vi "MODBUS_read_register.vi"(5 "Byte order":T1(ring)=enum."2-3-0-1", 6 "data type":enum16{"float", "UINT", "UINT32", "STRING"}(ring)=enum."STRING", 7 "MODBUS Serial Parameters":T3={"Mode"=enum."RTU", "Default Slave Address"=111, "MODBUS timeout"=1000, "Baud Rate"=38400, "Parity"=0, "Flow Control"=0} {"Parity" items=["None", "Odd", "Even", "Mark", "Space"]; "Flow Control" items=["None", "XON/XOFF", "RTS/CTS", "XON/XOFF & RTS/CTS", "DTR/DSR", "XON/XOFF & DTR/DSR"]}, 8 "error in":errorcluster, 9 "Register":u16=285, 10 "Length":u16=1, 11 "VISA resource name":refnum<visa-resource-name>="MODBUS_485") -> (0 "error out":errorcluster, 1 "found?":bool, 2 "output cluster":T2, 3 "VISA resource name out":refnum<visa-resource-name>)   [LabVIEW 2016]
uses:
  NI Modbus.llb/MB Serial Master Query Read Holding Registers (poly).vi
  Manthey ModBus.llb/03 Read output registers.vi
panel:
  out "string out":string
  out "float out":sgl=496.2269
  out "U32 out":u32
  out "U16 out":u16
  out "Error Message":string
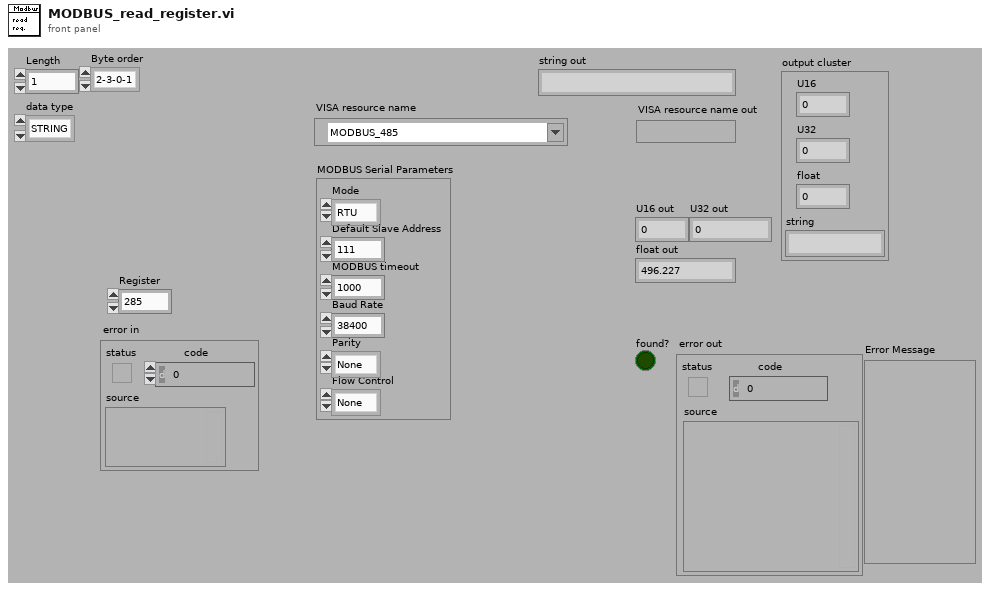
[diagram p1: front panel]
types:
  T1 = enum16{"0-1-2-3", "2-3-0-1", "1-0-3-2", "3-2-1-0"}
  T2 = cluster{"U16":u16, "U32":u32, "float":sgl, "string":string}
  T3 = cluster{"Mode":enum16{"RTU", "ASCII"}, "Default Slave Address":u8, "MODBUS timeout":u32, "Baud Rate":u32, "Parity":u16, "Flow Control":u16}
  T4 = cluster{"Mode":enum16{"RTU", "ASCII"}, "Default Slave Address":u8}
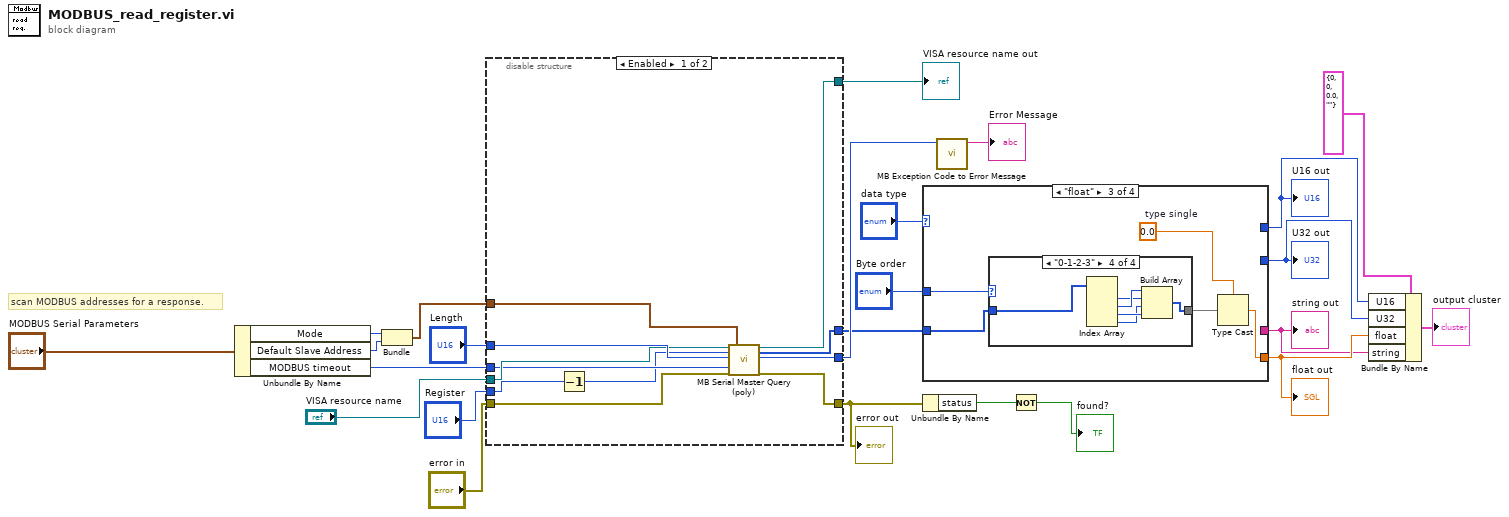
[diagram p0: block diagram]
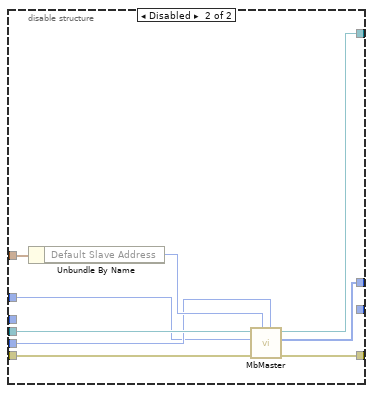
[diagram p2: hidden frame]
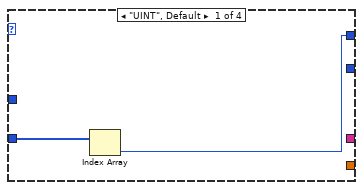
[diagram p3: hidden frame]
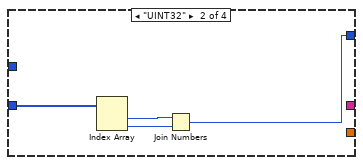
[diagram p4: hidden frame]
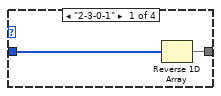
[diagram p5: hidden frame]
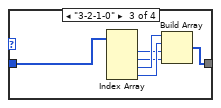
[diagram p7: hidden frame]
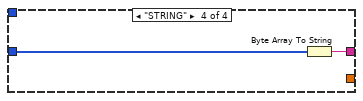
[diagram p8: hidden frame]
diagram:
  # "scan MODBUS addresses for a response."
  n1 = Unbundle By Name("MODBUS Serial Parameters") -> ("Mode"=w13:enum16{"RTU", "ASCII"}, "Default Slave Address"=w12:u8, "MODBUS timeout"=w10:u32)
  n2 = Bundle("Mode"=w13, "Default Slave Address"=w12) -> (w11:T4)  [unwired: 1 in]
  n3 = disable-structure shown="Enabled" {
    disable-tunnel: [w35 w39] -> w23
    disable-tunnel: [w34 w41] -> w22
    disable-tunnel: [w33 _] -> w19
    disable-tunnel: "Register" -> [w26 w37]
    disable-tunnel: "Length" -> [w32 w36]
    disable-tunnel: [w31 w40] -> w2
    disable-tunnel: "VISA resource name" -> [w30 w42]
    disable-tunnel: "error in" -> [w29 w38]
    disable-tunnel: w11 -> [w28 w44]
    disable-tunnel: w10 -> [w27 _]
    frame Enabled {
      n4 = Decrement(x=w26) -> (x-1=w25:u16)
      n5 = call-poly "MB Serial Master Query (poly).vi"("VISA resource name"=w30, "Starting Address"=w25, "Quantity"=w32, "Timeout"=w27, "error in"=w29, "Serial Parameters"=w28) -> ("VISA resource name out"=w34:refnum<visa-resource-name>, "Holding Registers"=w31:u16[], "Exception Code"=w33:u8, "error out"=w35:errorcluster)  [unwired: 10 out]
    }
    frame Disabled {
      n6 = Unbundle By Name(w44) -> ("Default Slave Address"=w43:u8)
      n7 = call-poly "MbMaster.vi"("Protocol Start Address"=w37, "Modbus Slave Address"=w43, "error in (no error)"=w38, "Number of Points"=w36, "VISA resource name"=w42) -> ("error out"=w39:errorcluster, "Array of Registers"=w40:u16[], "VISA resource name out"=w41:refnum<visa-resource-name>)  [unwired: 3 in, 1 out]
    }
  }
  "error out" <- w23
  "VISA resource name out" <- w22
  n8 = case shown="\"float\"" "data type" {
    tunnel: w2 -> [w46 w50 w53 w72]
    tunnel: [w45 _ _ _] -> w16
    tunnel: [_ w47 _ _] -> w15
    tunnel: [_ _ w54 _] -> w14
    tunnel: [_ _ _ w71] -> w4
    tunnel: "Byte order" -> [_ _ w51 _]
    frame "UINT", Default {
      n9 = Index Array(array=w46) -> (element=w45:u16)  [unwired: 1 in]
    }
    frame "UINT32" {
      n10 = Index Array(array=w50) -> (element #1=w49:u16, element #2=w48:u16)  [unwired: 2 in]
      n11 = Join Numbers(hi=w49, lo=w48) -> ((hi.lo)=w47:u32)
    }
    frame "float" {
      w55 = sgl 0.0  # type single
      n12 = case shown="\"0-1-2-3\"" w51 {
        tunnel: w53 -> [w57 w58 w64 w70]
        tunnel: [w56 w58 w59 w69] -> w52
        frame "2-3-0-1" {
          n13 = Reverse 1D Array(array=w57) -> (reversed array=w56:u16[])
        }
        frame "1-0-3-2" {
        }
        frame "3-2-1-0" {
          n14 = Index Array(array=w64) -> (element #1=w61:u16, element #2=w60:u16, element #3=w63:u16, element #4=w62:u16)  [unwired: 4 in]
          n15 = Build Array(w63, w62, w61, w60) -> (w59:u16[])
        }
        frame "0-1-2-3" {
          n16 = Index Array(array=w70) -> (element #1=w67:u16, element #2=w68:u16, element #3=w66:u16, element #4=w65:u16)  [unwired: 4 in]
          n17 = Build Array(w68, w67, w65, w66) -> (w69:u16[])
        }
      }
      n18 = Type Cast(type=w55, x=w52) -> (*(type *) &x=w54:sgl)
    }
    frame "STRING" {
      n19 = Byte Array To String(unsigned byte array=w72) -> (string=w71:string)
    }
  }
  "U16 out" <- w16
  "U32 out" <- w15
  "float out" <- w14
  "string out" <- w4
  n20 = Unbundle By Name(w23) -> ("status"=w21:bool)
  n21 = call "MB Exception Code to Error Message.vi"("Exception Code"=w19) -> ("Error Message"=→"Error Message":string)  [unwired: 10 in]
  n22 = Not(x=w21) -> (.not. x?=→"found?":bool)
  n23 = Bundle By Name(cluster=T2 {"U16"=0, "U32"=0, "float"=0.0, "string"=""} ("output cluster"), "U16"=w16, "U32"=w15, "float"=w14, "string"=w4) -> (→"output cluster":T2)
